vi "Cxns-Endpoints To Outputs.vi"(0 "Connection File Path":path, 2 "Section":string, 7 "Endpoints":string[](array[string]), 11 "error in (no error)":errorcluster) -> (8 "Outputs":i32[](array[numeric]), 15 "error out":errorcluster)   [LabVIEW 2015]
uses:
  <vilib>/Utility/config.llb/Read Key (String).vi
  <vilib>/Utility/config.llb/NI_LVConfig.lvlib
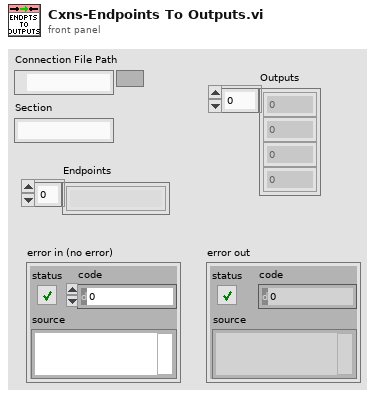
[diagram p1: front panel]
types:
  T1 = typedef "NI_LVConfig.lvlib/Config Data RefNum.ctl" = refnum<k1>
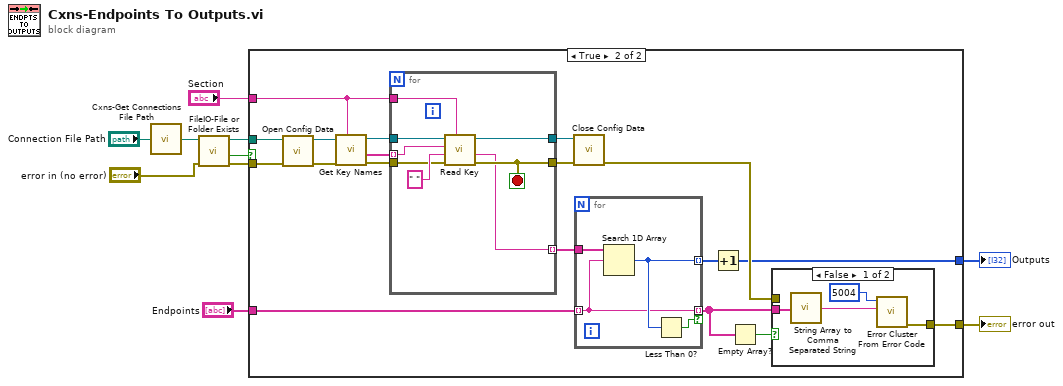
[diagram p0: block diagram]
diagram:
  n1 = call "Cxns-Get Connections File Path.vi"("Connection File Path"="Connection File Path") -> ("Path Out"=w9:path)
  n2 = call "FileIO-File or Folder Exists.vi"("error in (no error)"="error in (no error)", "path"=w9) -> ("error out"=w5:errorcluster, "Exists?"=w7:bool, "dup path"=w6:path)  [unwired: 6 in, 1 out]
  n3 = case shown="True" w7 {
    tunnel: w6 -> [_ w29]
    tunnel: w5 -> [w11 w28]
    tunnel: "Section" -> [_ w23]
    tunnel: [w11 w15] -> w3
    tunnel: "Endpoints" -> [_ w17]
    tunnel: [_ w12] -> w1
    frame False {
    }
    frame True {
      n4 = call <vilib>:"Open Config Data.vi"("error in (no error)"=w28, "configuration file path"=w29) -> ("error out"=w26:errorcluster, "refnum"=w27:T1)  [unwired: 7 in, 1 out]
      n5 = call <vilib>:"Get Key Names.vi"("section"=w23, "error in (no error)"=w26, "refnum"=w27) -> ("error out"=w22:errorcluster, "key names"=w24:string[], "refnum out"=w25:T1)  [unwired: 5 in, 1 out]
      n6 = for {
        tunnel: w25 -> [w42]
        tunnel: w24 -> [w36] mode=indexing
        tunnel: [w40] -> w20
        tunnel: w23 -> [w39]
        tunnel: [w35] -> w19 mode=indexing
        tunnel: w22 -> [w38]
        tunnel: [w37] -> w21
        stop <- w37 stop-if-true
        n7 = call-poly <vilib>:"Read Key.vi"("section"=w39, "error in (no error)"=w38, "default value"=" ", "key"=w36, "refnum"=w42) -> ("error out"=w37:errorcluster, "value"=w35:string, "refnum out"=w40:T1)  [unwired: 3 in, 1 out]
      }
      n8 = call <vilib>:"Close Config Data.vi"("error in (no error)"=w21, "refnum"=w20) -> ("error out"=w16:errorcluster)  [unwired: 8 in, 1 out]
      n9 = for {
        tunnel: w17 -> [w44] mode=indexing
        tunnel: w19 -> [w46]
        tunnel: [w45] -> w18 mode=indexing
        tunnel: [w44] -> w13 mode=indexing if=w43
        n10 = Search 1D Array(1D array=w46, element=w44) -> (index of element=w45:i32)  [unwired: 1 in]
        n11 = Less Than 0?(x=w45) -> (x < 0?=w43:bool)
      }
      n12 = Increment(x=w18) -> (x+1=w12:i32[])
      n13 = Empty Array?(array=w13) -> (empty?=w14:bool)
      n14 = case shown="False" w14 {
        tunnel: w16 -> [_ w34]
        tunnel: [w32 w34] -> w15
        tunnel: w13 -> [w33 _]
        frame False {
          n15 = call "String Array to Comma Separated String.vi"("String Array"=w33) -> ("comma separated string"=w31:string)
          n16 = call <vilib>:"Error Cluster From Error Code.vi"("error message (\"\")"=w31, "error code (0)"=5004) -> ("error out"=w32:errorcluster)  [unwired: 7 in]
        }
        frame True {
        }
      }
    }
  }
  "error out" <- w3
  "Outputs" <- w1
